vi "ArrayToImage.vi"() -> ()   [LabVIEW 2017]
panel:
  out "output array":dbl[][](array[numeric])
  in  "Rows":i32=64
  in  "Columns":i32=64
  out "Image":T1(plugin-control)
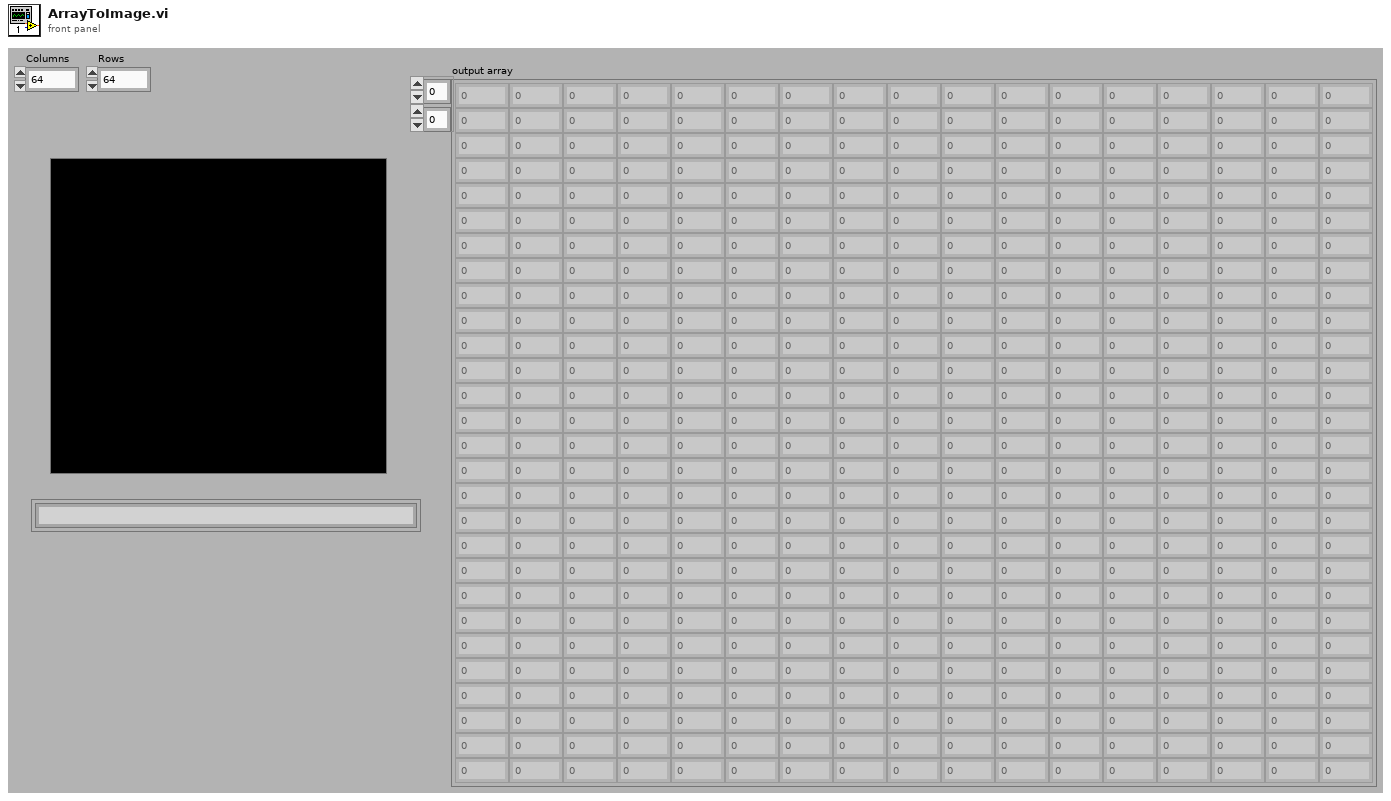
[diagram p1: front panel]
types:
  T1 = typedef "IMAQ Image.ctl" = refnum<image>
  T2 = typedef "Image Type" = u32
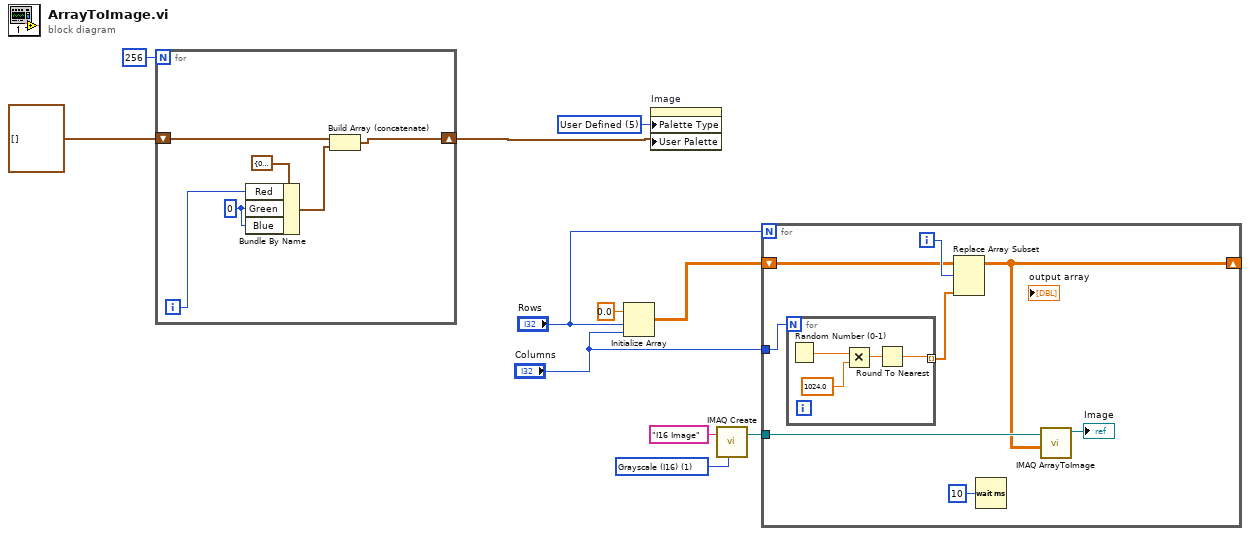
[diagram p0: block diagram]
diagram:
  w4 = u32 5 items=["Grayscale", "Binary", "Gradient", "Rainbow", "Temperature", "User Defined", "Binary 16 Bit", "Gradient 16 Bit", "Rainbow 16 Bit", "Temperature 16 Bit", "User Defined 16 Bit"] ("Palette:Palette Type")
  w10 = T2 1 items=["Grayscale (U8)", "Grayscale (I16)", "Grayscale (SGL)", "Complex (CSG)", "RGB (U32)", "HSL (U32)", "RGB (U64)"] ("Image Type")
  n1 = for {
    N: 256 -> [_]
    shift-right: [w15] -> w1
    shift-left: cluster{"Red":u8, "Green":u8, "Blue":u8}[] [] ("Palette:User Palette") -> [w16]
    i -> [w13]
    w12 = u8 0 ("Green")
    n2 = Bundle By Name(cluster=cluster{"Red":u8, "Green":u8, "Blue":u8} {"Red"=0, "Green"=0, "Blue"=0}, "Red"=w13, "Green"=w12, "Blue"=w12) -> (w14:cluster{"Red":u8, "Green":u8, "Blue":u8})
    n3 = Build Array (concatenate)(w16, w14) -> (w15:cluster{"Red":u8, "Green":u8, "Blue":u8}[])
  }
  n4 = Initialize Array(0.0 ("element"), "Rows", "Columns") -> (w6:dbl[][])
  n5 = property on="Image" class="ImageControl"("Palette Type"=w4, "User Palette"=w1) -> ()  [unwired: 2 in, 2 out]
  n6 = call "IMAQ Create"("Image Name"="I16 Image", "Image Type"=w10) -> ("New Image"=w5:T1)  [unwired: 3 in, 1 out]
  n7 = for {
    N: "Rows" -> [_]
    tunnel: "Columns" -> [w25]
    tunnel: w5 -> [w21]
    shift-right: [w18] -> _
    shift-left: w6 -> [w19]
    i -> [w24]
    n8 = for {
      N: w25 -> [_]
      tunnel: [w26] -> w23 mode=indexing
      n9 = Random Number (0-1)() -> (number: 0 to 1=w29:dbl)
      n10 = Multiply(x=w29, y=1024.0) -> (x*y=w27:dbl)
      n11 = Round To Nearest(number=w27) -> (nearest integer value=w26:dbl)
    }
    n12 = Replace Array Subset(array=w19, new element=w23, index (row)=w24) -> (w18:dbl[][])  [unwired: 1 in]
    n13 = Wait (ms)(milliseconds to wait=u32 10) -> ()  [unwired: 1 out]
    n14 = call "IMAQ ArrayToImage"("Image Pixels (I16)"=w18, "Image"=w21) -> ("Image Out"=→"Image":T1)  [unwired: 8 in, 1 out]
  }
